vi "Flush Data to Log File.vi"(8 "error in (no error)":errorcluster, 10 "Data Queue":T1, 11 "Logging Configuration":T2) -> (0 "error out":errorcluster)   [LabVIEW 2018, in "Logging.lvlib"]
doc: "Flush the data queue of any pending data and write it to the log file. Close the TDMS file reference."
uses:
  Logging.lvlib
  Logging Configuration.ctl
  <vilib>/addons/database/Connection.llb/Conn ObjectReference.ctl
  Controls/Data Queue.ctl
  Controls/Acquired Data.ctl
  <vilib>/addons/database/NI_Database_API.lvlib
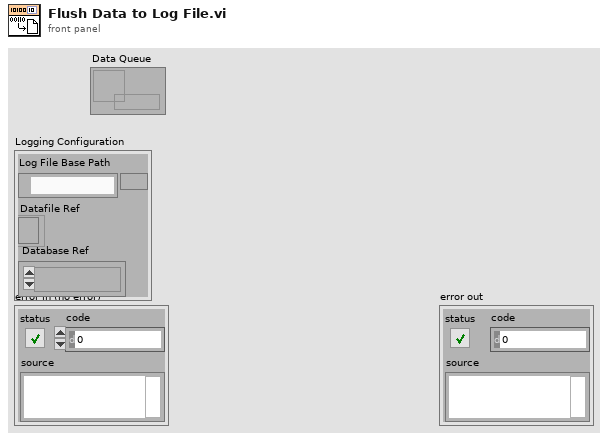
[diagram p1: front panel]
types:
  T1 = typedef "Data Queue.ctl" = refnum<queue>
  T2 = typedef "Logging.lvlib/Logging Configuration.ctl" = cluster{"Log File Base Path":path, "Datafile Ref":refnum<file>, "Database Ref":T3}
  T3 = typedef "NI_Database_API.lvlib/Conn ObjectReference.ctl" = refnum<k1>
  T4 = typedef "Acquired Data.ctl" = cluster{"offset":dbl, "time":string}
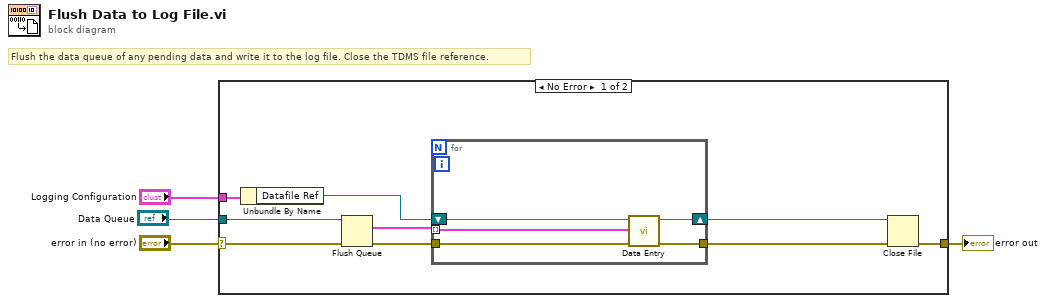
[diagram p0: block diagram]
diagram:
  # "Flush the data queue of any pending data and write it to the log file. Close the TDMS file reference."
  n1 = case shown="No Error" "error in (no error)" {
    selector: "error in (no error)" -> [w7 w19]
    tunnel: "Data Queue" -> [w11 _]
    tunnel: "Logging Configuration" -> [w10 _]
    tunnel: [w8 w19] -> w3
    frame No Error {
      n2 = Unbundle By Name(w10) -> ("Datafile Ref"=w12:refnum<file>)
      n3 = Flush Queue(queue=w11, error in (no error)=w7) -> (remaining elements=w13:T4[], error out=w6:errorcluster)  [unwired: 1 out]
      n4 = for {
        shift-right: [w17] -> w9
        shift-left: w12 -> [w18]
        tunnel: w13 -> [w16] mode=indexing
        tunnel: w6 -> [w15]
        tunnel: [w14] -> w5
        n5 = call "Data Entry.vi"("error in (no error)"=w15, "Data"=w16, "Byte Stream File in"=w18) -> ("error out"=w14:errorcluster, "Byte Stream File out"=w17:refnum<file>)  [unwired: 7 in]
      }
      n6 = Close File(refnum=w9, error in=w5) -> (error out=w8:errorcluster)  [unwired: 1 out]
    }
    frame Error {
    }
  }
  "error out" <- w3
